vi "Create Error File.vi"(11 "File Contents":string) -> (3 "Filename":string)   [LabVIEW 2013]
uses:
  Error File Queue Contents.ctl
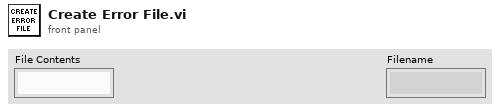
[diagram p1: front panel]
types:
  T1 = typedef "Error File Queue Contents.ctl" = cluster{"Filename":string, "File Contents":string, "Time Stamp":timestamp, "Origin":string}
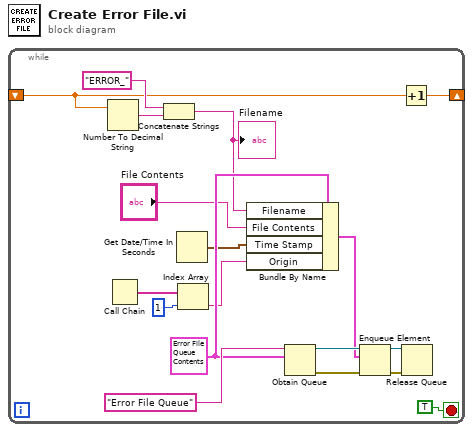
[diagram p0: block diagram]
diagram:
  n1 = while {
    shift-right: [w5] -> _
    shift-left: _ -> [w6]
    stop <- TRUE stop-if-true
    w13 = T1 {"Filename"="", "File Contents"="", "Time Stamp"=timestamp(0 s since 1904-01-01), "Origin"=""} ("Cluster")
    n2 = Number To Decimal String(number=w6) -> (decimal integer string=w9:string)  [unwired: 1 in]
    n3 = Call Chain() -> (call chain=w4:string[])
    n4 = Concatenate Strings("ERROR_" ("string"), w9) -> (w7:string)
    "Filename" <- w7
    n5 = Get Date/Time In Seconds() -> (seconds since 1Jan1904=w10:timestamp)
    n6 = Index Array(array=w4, index=1) -> (element=w2:string)
    n7 = Bundle By Name(cluster=w13, "Filename"=w7, "File Contents"="File Contents", "Time Stamp"=w10, "Origin"=w2) -> (w1:T1)
    n8 = Obtain Queue(name (unnamed)="Error File Queue", element data type=w13) -> (queue out=w18:refnum<queue>, error out=w16:errorcluster)  [unwired: 3 in, 1 out]
    n9 = Enqueue Element(queue=w18, element=w1, error in (no error)=w16) -> (queue out=w17:refnum<queue>, error out=w15:errorcluster)  [unwired: 1 in, 1 out]
    n10 = Increment(x=w6) -> (x+1=w5:dbl)
    n11 = Release Queue(queue=w17, error in (no error)=w15) -> ()  [unwired: 1 in, 3 out]
  }
